vi "Set Icon Body Text.vi"(8 "error in (no error)":errorcluster, 10 "Body Text":T1 {"Body Text Spec"."Alignment" items=["left", "center", "right"]}, 11 "VI Path":string) -> (0 "error out":errorcluster)   [LabVIEW 2013]
uses:
  <vilib>/LabVIEW Icon API/lv_icon/Controls/BodyText.ctl
  <vilib>/LabVIEW Icon API/lv_icon/Controls/Font.ctl
  <vilib>/LabVIEW Icon API/lv_icon/Controls/Alignment.ctl
  <vilib>/LabVIEW Icon API/lv_icon/Classes/Icon/Icon.lvclass
  <vilib>/LabVIEW Icon API/lv_icon/Classes/Icon Framework/Icon Framework.lvclass
  <vilib>/LabVIEW Icon API/LabVIEW Icon API.lvlib
panel:
  out "VI Path (dup)":string
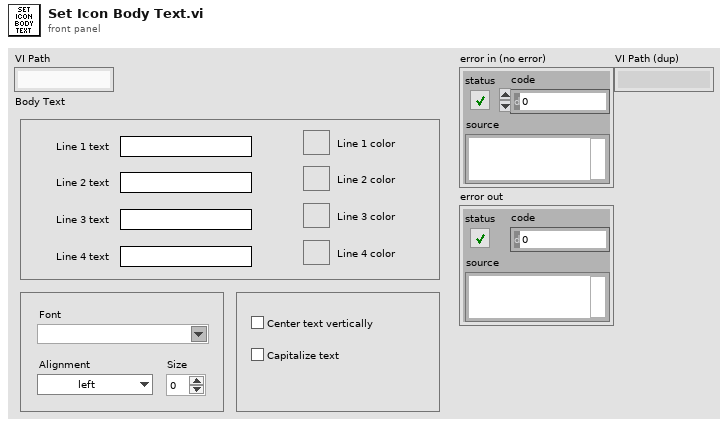
[diagram p1: front panel]
types:
  T1 = typedef "BodyText.ctl" = cluster{"Line 1 text":string, "Line 2 text":string, "Line 3 text":string, "Line 4 text":string, "Line 1 color":u32, "Line 2 color":u32, "Line 3 color":u32, "Line 4 color":u32, "Body Text Spec":cluster{"Font":T2, "Alignment":T3, "Size":u8}, "Center text vertically":bool, "Capitalize Text":bool}
  T2 = typedef "Font.ctl" = string
  T3 = typedef "Alignment.ctl" = u16
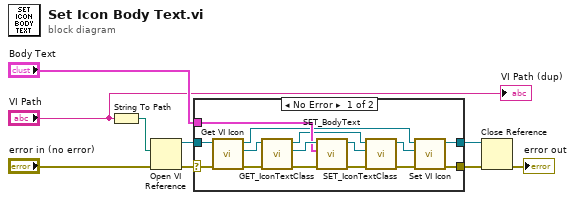
[diagram p0: block diagram]
diagram:
  n1 = String To Path(string="VI Path") -> (path=w1:path)
  n2 = Open VI Reference(vi path=w1, error in (no error)="error in (no error)") -> (vi reference=w8:refnum<vi>, error out=w9:errorcluster)  [unwired: 4 in]
  n3 = case shown="No Error" w9 {
    selector: w9 -> [w23 w25]
    tunnel: w8 -> [w24 w26]
    tunnel: [w11 w25] -> w6
    tunnel: [w10 w26] -> w7
    tunnel: "Body Text" -> [w19 _]
    frame No Error {
      n4 = call <vilib>:"Get VI Icon.vi"("error in (no error)"=w23, "VI Refnum in"=w24) -> ("error out"=w22:errorcluster, "Icon"=w21:refnum<class "Icon.lvclass">, "VI Refnum out"=w14:refnum<vi>)  [unwired: 7 in]
      n5 = call-dynamic "GET_IconTextClass.vi"("error in (no error)"=w22, "Icon.lvclass in"=w21) -> ("error out"=w16:errorcluster, "Icon Framework.lvclass"=w20:refnum<class "Icon Framework.lvclass">, "Icon.lvclass out"=w18:refnum<class "Icon.lvclass">)  [unwired: 7 out]
      n6 = call-dynamic "SET_BodyText.vi"("error in (no error)"=w16, "Body Text"=w19, "Icon Framework.lvclass in"=w20) -> ("error out"=w15:errorcluster, "Icon Framework.lvclass out"=w17:refnum<class "Icon Framework.lvclass">)  [unwired: 7 in]
      n7 = call-dynamic "SET_IconTextClass.vi"("error in (no error)"=w15, "Icon Framework.lvclass"=w17, "Icon.lvclass in"=w18) -> ("error out"=w12:errorcluster, "Icon.lvclass out"=w13:refnum<class "Icon.lvclass">)  [unwired: 7 in]
      n8 = call <vilib>:"Set VI Icon.vi"("error in (no error)"=w12, "Icon"=w13, "VI Refnum in"=w14) -> ("error out"=w11:errorcluster, "VI Refnum out"=w10:refnum<vi>)  [unwired: 7 in]
    }
    frame Error {
    }
  }
  n9 = Close Reference(reference=w7, error in (no error)=w6) -> (error out=→"error out":errorcluster)
  "VI Path (dup)" <- "VI Path"
